vi "Generate.vi"(0 "reference in":refnum<class "Scripting.lvclass">, 1 "Path":path, 3 "Classes":T1[](array[typedef]), 5 "error in (no error)":errorcluster) -> (14 "reference out":refnum<class "Scripting.lvclass">, 19 "error out":errorcluster)   [LabVIEW 2018, in "Scripting.lvclass"]
uses:
  Scripting.lvclass
  Executer_class/typedefs/ClassDescription.ctl
  Executer_class/typedefs/MethodDescription.ctl
  Executer_class/Executer.lvclass
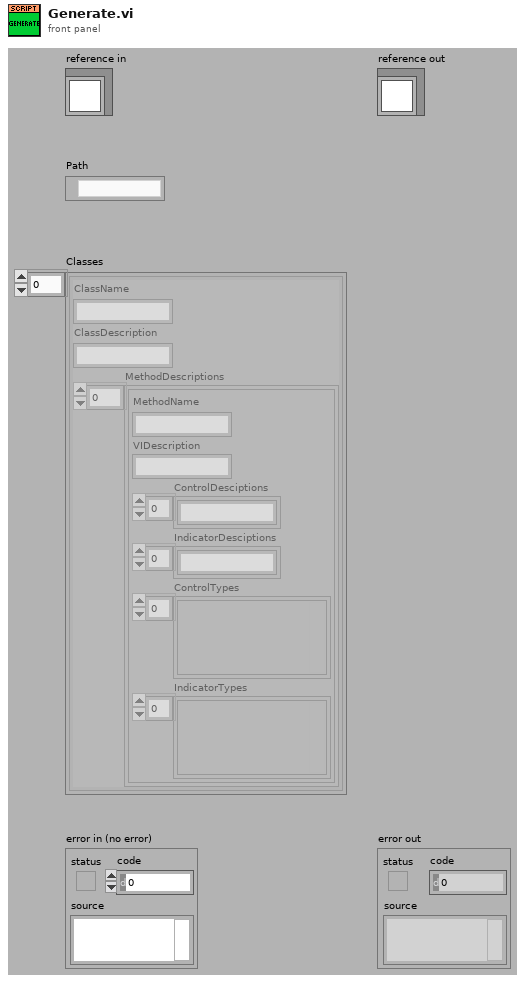
[diagram p1: front panel]
types:
  T1 = typedef "Executer.lvclass/ClassDescription.ctl" = cluster{"ClassName":string, "ClassDescription":string, "MethodDescriptions":T2[]}
  T2 = typedef "Executer.lvclass/MethodDescription.ctl" = cluster{"MethodName":string, "VIDescription":string, "ControlDesciptions":string[], "IndicatorDesciptions":string[], "ControlTypes":variant[], "IndicatorTypes":variant[]}
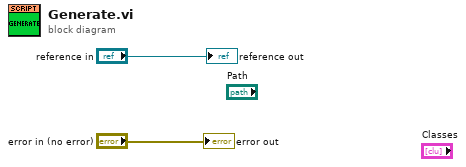
[diagram p0: block diagram]
diagram:
  "error out" <- "error in (no error)"
  "reference out" <- "reference in"
